vi "Init.vi"(8 "error in (no error)":errorcluster, 10 "Connection":T1={"Client ID"="LabVIEW_MQTT_Client", "Host"="", "Port"=1883, "Connection Timeout"=2000, "Write Timeout"=2000, "Read Timeout"=2000, "Sub Timeout"=30000, "Keep Alive (sec)"=60, "Clean Session"=FALSE}, 11 "MQTT in":refnum<class "MQTT Client.lvclass">) -> (0 "error out":errorcluster, 3 "MQTT out":refnum<class "MQTT Client.lvclass">)   [LabVIEW 2020, in "MQTT Client.lvclass"]
uses:
  MQTT Client.lvclass
  mqttTypedef/ConnectionConfig.ctl
  mqttCmd/BaseMqttMsg.lvclass
  MQTT Client.lvclass/MQTT Client.ctl
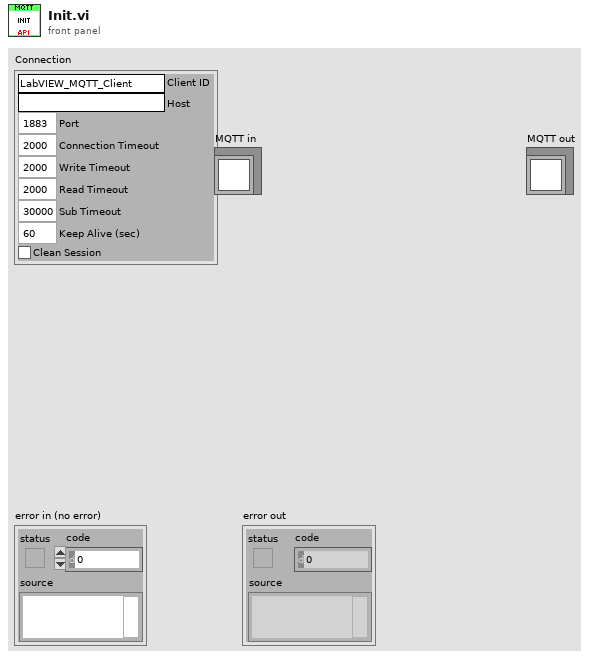
[diagram p1: front panel]
types:
  T1 = typedef "MQTT Client.lvclass/ConnectionConfig.ctl" = cluster{"Client ID":string, "Host":string, "Port":u16, "Connection Timeout":i32, "Write Timeout":i32, "Read Timeout":i32, "Sub Timeout":i32, "Keep Alive (sec)":u16, "Clean Session":bool}
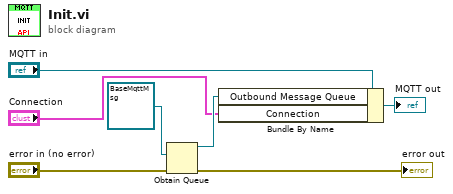
[diagram p0: block diagram]
diagram:
  n1 = Obtain Queue(element data type=refnum<class "BaseMqttMsg.lvclass"> refnum ("BaseMqttMsg.lvclass"), error in (no error)="error in (no error)") -> (queue out=w3:refnum<queue>, error out=→"error out":errorcluster)  [unwired: 3 in, 1 out]
  n2 = Bundle By Name(cluster="MQTT in", "Outbound Message Queue"=w3, "Connection"="Connection") -> (→"MQTT out":refnum<class "MQTT Client.lvclass">)
